vi "Get Channel Units.vi"(10 "Log Units":bool, 11 "TDMS Channel Info":T1) -> (3 "Unit String Out":string[](array[string]))   [LabVIEW 2022 SP3, in "CSV Export.lvlib" / "CSV Export.lvclass"]
uses:
  CSV Export.lvclass
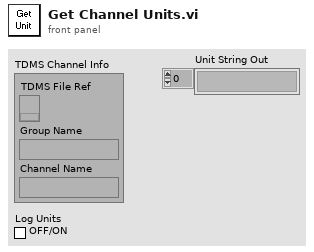
[diagram p1: front panel]
types:
  T1 = cluster{"TDMS File Ref":refnum<k34>, "Group Name":string, "Channel Name":string}
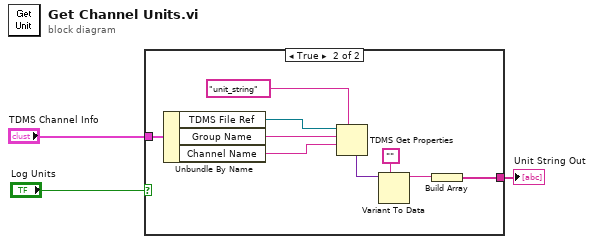
[diagram p0: block diagram]
diagram:
  n1 = case shown="True" "Log Units" {
    tunnel: "TDMS Channel Info" -> [_ w12]
    tunnel: [_ w4] -> w1
    frame False {
    }
    frame True {
      n2 = Unbundle By Name(w12) -> ("TDMS File Ref"=w11:refnum<k34>, "Group Name"=w10:string, "Channel Name"=w9:string)
      n3 = TDMS Get Properties(7:"unit_string", 9:w9, 10:w10, 11:w11) -> (4:w7:variant)  [unwired: 2 in, 5 out]
      n4 = Variant To Data(type="", Variant=w7) -> (data=w5:string)  [unwired: 1 in, 1 out]
      n5 = Build Array(w5) -> (w4:string[])
    }
  }
  "Unit String Out" <- w1
